vi "DAC_wave_ouput.vi"() -> ()   [LabVIEW 2010]
uses:
  libdaqVI.lvlib
  <vilib>/measure/NI_MABase.lvlib
panel:
  out "波形图":waveform(dbl)(graph)
  in  "DAC通道选择":enum16{"DAC1", "DAC2"}(ring)
  in  "波形重复次数":u32
  in  "exit":bool
  in  "dac output":bool
  in  "波形采样点数":dbl=10.0
  in  "采样频率(Hz)":dbl=10000.0 format="%#_6p"
  in  "square wave duty cycle (%)":dbl=50.0 caption="方波占空比(%)" format="%0.2f"
  in  "offset":dbl=1.0 caption="直流偏移量(V)" format="%0.2p"
  in  "signal type":T1(ring) caption="信号类型"
  in  "phase":dbl caption="相位(度)" format="%.2p"
  in  "amplitude":dbl=1.0 caption="幅值(V)" format="%0.2p"
  in  "frequency":dbl=1000.0 caption="频率(Hz)" format="%0.2p"
  out "采集卡状态":bool
  out "设备名称":string
  out "设备数量":u32
  # "范例说明：\n1、范例演示了如何调用API通过DAC模块输出波形，可以输出正弦波、三角波、锯齿波和方波四种波形；该范例支持的采集卡有：DAQ-USB3212、DAQ-USB3213、DAQ-USB3214\nDAQ-USB3212 量程:0-5V\nDAQ-USB3213 量程:0-10V\nDAQ-USB3214 量程:±10V\n2、运行程序之后，设置波形生成参数和波形输出参数，选择输出的DAC通道，再点击“波形输出”，在右侧波形图中可看到生成的波形；\n3、注意：DAQ-USB3212、DAQ-USB3213不支持负压输出，因此波形需要增加直流偏移量，否则负压部分会截断；根据经验正弦信号采样率一般需要设置为波形频率的10倍以上，锯齿波、三角波、方波一般需要设置为波形频率的20倍以上，才能较好的还原信号。"
  # "DAQ-DAC波形输出演示程序"
  # "波形生成设置"
  # "波形输出设置"
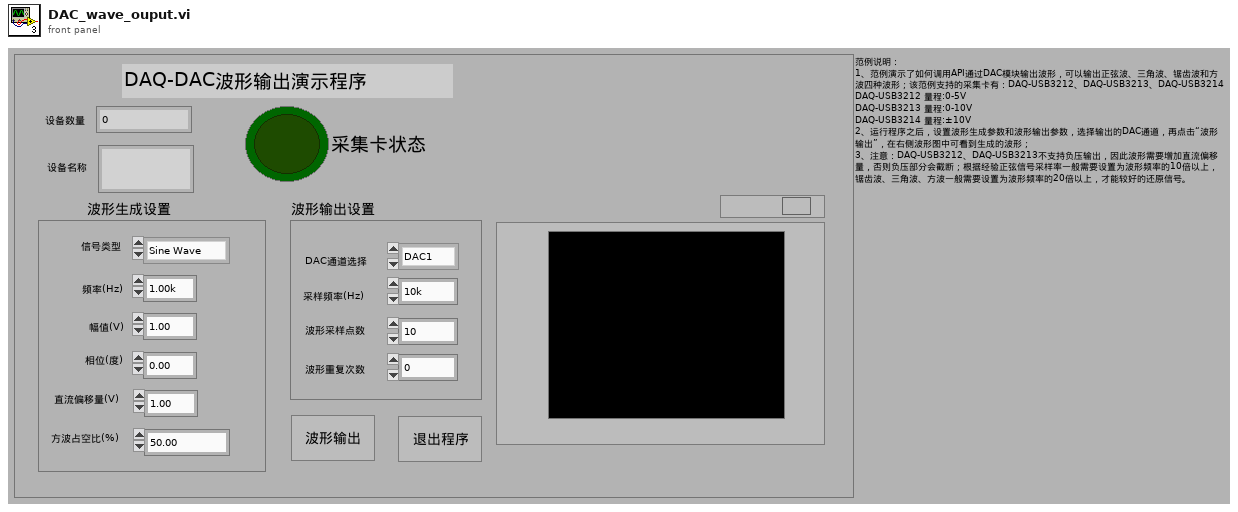
[diagram p1: front panel]
types:
  T1 = enum16{"Sine Wave", "Triangle Wave", "Square Wave", "Sawtooth Wave"}
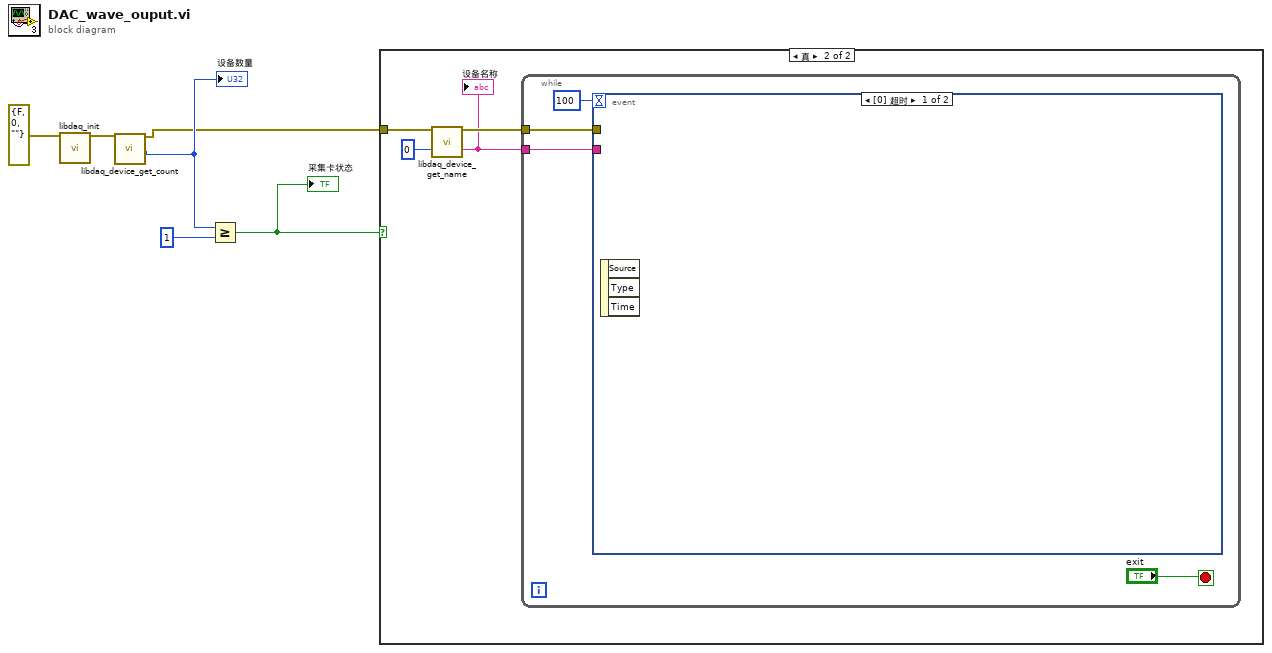
[diagram p0: block diagram]
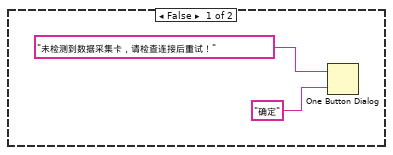
[diagram p2: hidden frame]
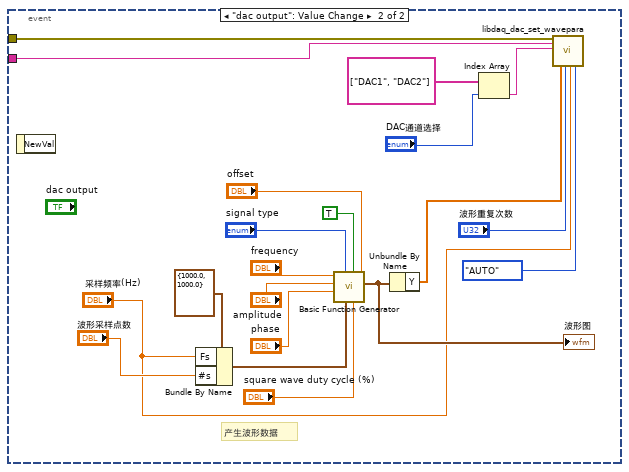
[diagram p3: hidden frame]
diagram:
  n1 = call "libdaq_init.vi"("error in (no error)"=errorcluster {"status"=FALSE, "code"=0, "source"=""}) -> ("error out"=w3:errorcluster)  [unwired: 18 in]
  n2 = call "libdaq_device_get_count.vi"("error in (no error)"=w3) -> ("error out"=w1:errorcluster, "device_count"=w2:i32)  [unwired: 17 in]
  "设备数量" <- w2
  n3 = Greater Or Equal?(x=w2, y=u32 1 ("name length")) -> (x >= y?=w5:bool)
  "采集卡状态" <- w5
  n4 = case shown="真" w5 {
    tunnel: w1 -> [_ w12]
    frame False {
      n5 = One Button Dialog(message="未检测到数据采集卡，请检查连接后重试！" ("消息"), button name ("OK")="确定" ("按钮名称（“确定”）")) -> ()  [unwired: 1 out]
    }
    frame True {
      n6 = call "libdaq_device_get_name.vi"("error in (no error)"=w12, "device_index"=u32 0 ("name length")) -> ("error out"=w10:errorcluster, "device_name"=w9:string)  [unwired: 16 in]
      "设备名称" <- w9
      n7 = while {
        tunnel: w10 -> [w16]
        tunnel: w9 -> [w15]
        stop <- "exit" stop-if-true
        n8 = event shown="[0] 超时" {
          selector: _ -> [_ _]
          dyn-events: _ -> [_ _]
          timeout: 100 -> [_ _]
          tunnel: w16 -> [_ w34]
          tunnel: w15 -> [_ w33]
          event Timeout {
            n9 = event-data() -> ()  [unwired: 1 in, 3 out]
          }
          event "dac output": Value Change {
            # "产生波形数据"
            n10 = event-data() -> ()  [unwired: 1 in, 1 out]
            n11 = Bundle By Name(cluster=cluster{"Fs":dbl, "#s":dbl} {"Fs"=1000.0, "#s"=1000.0} ("sampling info"), "Fs"="采样频率(Hz)", "#s"="波形采样点数") -> (w31:cluster{"Fs":dbl, "#s":dbl})
            n12 = call <vilib>:"Basic Function Generator.vi"("offset"="offset", "square wave duty cycle (%)"="square wave duty cycle (%)", "reset signal"=TRUE, "sampling info"=w31, "signal type"="signal type", "phase"="phase", "amplitude"="amplitude", "frequency"="frequency") -> ("signal out"=w21:waveform(dbl))  [unwired: 1 in, 2 out]
            "波形图" <- w21
            n13 = Unbundle By Name(w21) -> ("Y"=w20:dbl[])
            n14 = Index Array(array=string[] ["DAC1", "DAC2"], index="DAC通道选择") -> (element=w35:string)
            n15 = call "libdaq_dac_set_wavepara.vi"("error in (no error)"=w34, "device_name"=w33, "module_name"=w35, "buf"=w20, "cycles"="波形重复次数", "frequency"="采样频率(Hz)", "trigger_mode"=enum16{"AUTO", "SOFT", "HARD"}."AUTO") -> ()  [unwired: 10 in, 3 out]
          }
        }
      }
    }
  }
